vi "Return_Data.vi"(8 "error in (no error)":errorcluster caption="entrée d'erreur (pas d'erreur)", 11 "Class Instrument Power_Supply en entrée":refnum<class "Class Instrument Power_Supply.lvclass">) -> (0 "error out":errorcluster caption="sortie d'erreur", 2 "Data_Json":string, 3 "Class Instrument Power_Supply en sortie":refnum<class "Class Instrument Power_Supply.lvclass">)   [LabVIEW 2020, in "Library Instrument & Equipement.lvlib" / "Library Instruments.lvlib" / "Class Instrument Power_Supply.lvclass"]
uses:
  Class Instrument Power_Supply.lvclass
  Class Instrument Power_Supply.lvclass/Class Instrument Power_Supply.ctl
  JSON API/Variant JSON/Variant to JSON.vi
  JSON API/JSON Value/Get Item by name array.vi
  JSON API/JSON Value/JSON Value.lvclass
  JSON API/Get Polymorphic/JSON GetSet.lvlib
  JSON API/Variant JSON/Variant JSON.lvlib
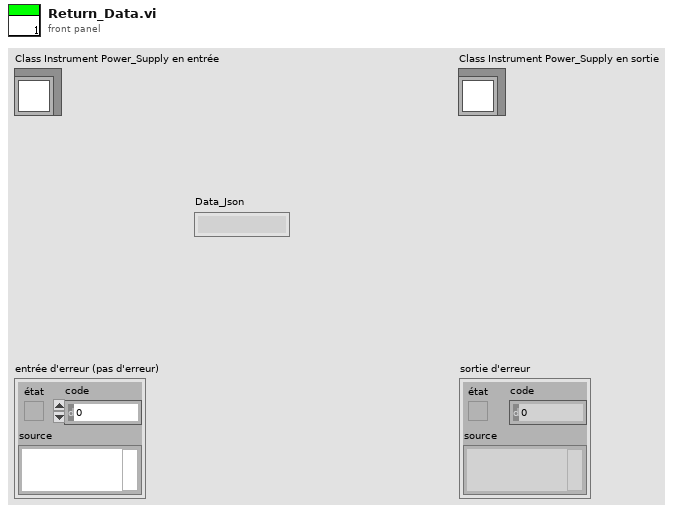
[diagram p1: front panel]
types:
  T1 = cluster{"Power":dbl, "Voltage":dbl, "Current":dbl}
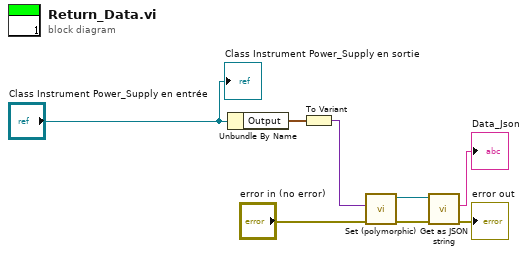
[diagram p0: block diagram]
diagram:
  n1 = Unbundle By Name("Class Instrument Power_Supply en entrée") -> ("Output"=w3:T1)
  n2 = To Variant(anything=w3) -> (Variant=w2:variant)
  n3 = call-poly "Set (polymorphic).vi"("error in (no error)"="error in (no error)", "Variant"=w2) -> ("error out"=w7:errorcluster, "JSON Value out"=w8:refnum<class "JSON Value.lvclass">)  [unwired: 8 in]
  n4 = call "Get as JSON string.vi"("error in (no error)"=w7, "JSON Value in"=w8) -> ("error out"=→"error out":errorcluster, "<JSON>"=→"Data_Json":string)  [unwired: 8 in]
  "Class Instrument Power_Supply en sortie" <- "Class Instrument Power_Supply en entrée"
